vi "2D Cartesian Coordinate Shift.vi"   [LabVIEW 2010, in "NI_AALPro.lvlib"]
doc: "Shifts two-dimensional Cartesian coordinates along the x- and y-axes. Wire data to the <B>X</B> input to determine the polymorphic instance to use or manually select the instance."
uses:
  NI_AALPro.lvlib
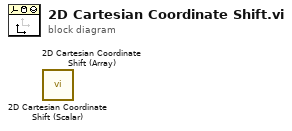
[diagram p0: block diagram]
diagram:
  n1 = call "2D Cartesian Coordinate Shift (Scalar).vi"() -> ()  [unwired: 9 in, 3 out]
  n2 = call "2D Cartesian Coordinate Shift (Array).vi"() -> ()  [unwired: 9 in, 3 out]
